vi "Ctrls state & value on Start-Stop.vi"(8 "error in (no error)":errorcluster, 11 "Queue data":T1) -> (0 "error out":errorcluster)   [LabVIEW 2020]
uses:
  Typedefs/Next state queue data.ctl
  Typedefs/Start-Stop Enum.ctl
  Typedefs/Top level VI states.ctl
  Typedefs/Read Write Enum.ctl
  Typedefs/Set Main VI cursor.ctl
  Global Variables/gl_UI Ctrl Refs.vi
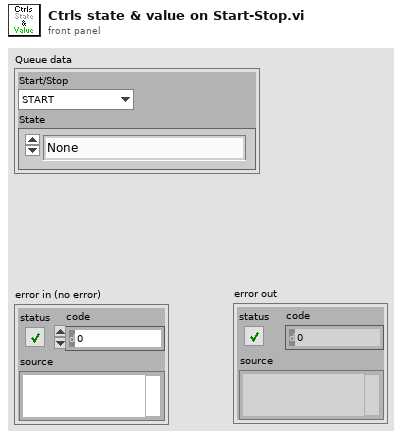
[diagram p1: front panel]
types:
  T1 = typedef "Next state queue data.ctl" = cluster{"Start/Stop":T2, "State":T3}
  T2 = typedef "Start-Stop Enum.ctl" = enum16{"START", "STOP"}
  T3 = typedef "Top level VI states.ctl" = enum16{"None", "Initialise UI", "<STACK PROTOCOL STATES>", "AOL Zstack-START", "AOL Zstack-STOP", "Motor Zstack-START", "Motor Zstack-STOP", "Parameter Sweep-START", "Parameter Sweep-STOP", "<ACQUISITION PROTOCOL STATES> ", "Functional Acquisition-START", "Functional Acquisition-STOP", "Single Plane Acquisition-START", "Single Plane Acquisition-STOP", "Volume Acquisition-START", "Volume Acquisition-STOP", "<LIVE IMAGING PROTOCOL STATES>", "Live Imaging-START", "Live Imaging-STOP", "Live Plane Imaging-START", "Live Plane Imaging-STOP", "Live Volume Imaging-START", "Live Volume Imaging-STOP", "<MOVEMENT CORRECTION PROTOCOL STATES>", "EXIT"}
  T4 = enum8{"Enabled", "Disabled", "Disabled and Grayed Out"}
  T5 = typedef "Read Write Enum.ctl" = enum16{"Read", "Write"}
  T6 = typedef "UI ctrl refs cluster.ctl" = cluster{"Top level VI path":path, "Top level VI ref":refnum<vi>, "User menu ref":refnum<k9>, "Sub Panel control":refnum<vi>, "Imaging Param Tab":refnum<vi>, "Occurrence-Start drivers":refnum<k4>, "Occurrence-Speed logging initialised":refnum<k4>, "Occurrence-XYZ stage initialised":refnum<k4>, "Exit button":refnum<vi>, "Status ind":refnum<vi>, "Set as origin":refnum<vi>, "Speed Logging":refnum<vi>, "Time Lapse":refnum<vi>, "Live Imaging":refnum<vi>, "AOL Z Stack":refnum<vi>, "Motor Z Stack":refnum<vi>, "Funct Acq button":refnum<vi>, "Hard Shutter":refnum<vi>, "Virtual Shutter":refnum<vi>, "Laser Power":refnum<vi>, "AOL Mode":refnum<vi>, "Frame Size":refnum<vi>, "Field of View":refnum<vi>, "Dwell Time":refnum<vi>, "Zoom":refnum<vi>, "AOL Z":refnum<vi>, "Objective":refnum<vi>, "Axis":refnum<vi>, "Paths & Names":refnum<vi>, "Experiment folder path (ind.)":refnum<vi>, "Last State (Ind.)":refnum<vi>, "Averages":refnum<vi>, "Angle (degrees)":refnum<vi>, "X centre":refnum<vi>, "Y centre":refnum<vi>, "Plane Mode":refnum<vi>, "# Planes":refnum<vi>, "Z Start":refnum<vi>, "Z Stop":refnum<vi>, "Z Step":refnum<vi>, "PMT 1":refnum<vi>, "PMT 2":refnum<vi>, "Stage XYZ Position":refnum<vi>, "Pockels@Z Start":refnum<vi>, "Pockels@Z Stop":refnum<vi>, "Obtain Z Start":refnum<vi>, "Obtain Z Stop":refnum<vi>, "Live stim.trig.period":refnum<vi>, "Live stim.trig.enable":refnum<vi>, "Movement Correction":refnum<vi>, "Load Reference Image":refnum<vi>, "XY Stage Move":refnum<vi>, "MovCor Cluster":refnum<vi>, "RefDAQParam":refnum<vi>, "Funct. Acq. Pockels Modulation":refnum<vi>, "Ref Laser Power":refnum<vi>, "Enable Video Recording":refnum<vi>, "Video Record-Live Imaging":refnum<vi>, "Video Record-Funct acq":refnum<vi>, "Reference Source":refnum<vi>, "AOL Z-stack Chirps Ready (ind)":refnum<vi>, "Target time between mov.cor. ref triggers (ms)":refnum<vi>, "Funct. Acq. Ref frame save":refnum<vi>, "Tracking button":refnum<vi>, "Show ref plots window":refnum<vi>, "Center freq ind (nm)":refnum<vi>, "Pickup mode (ind)":refnum<vi>, "Logging queue (ind)":refnum<vi>, "Back aperture power (ind.)":refnum<vi>, "Power after objective (ind.)":refnum<vi>, "Switch user":refnum<vi>, "Ls1 Conn. Status":refnum<vi>, "Ls1Tuning Status":refnum<vi>, "Ls1 Faults":refnum<vi>, "Ls1 Connection":refnum<vi>, "Ls1 Mode":refnum<vi>, "Ls1 POWER [mW]":refnum<vi>, "Ls1Shutter":refnum<vi>, "Ls1 Wavelength":refnum<vi>, "Ls1 Note":refnum<vi>, "Ls1 Confirm Wav":refnum<vi>, "Ls1 PreChrp Prism1":refnum<vi>, "Ls1 PreChrp Prism2":refnum<vi>, "Ls1 wav top Ind":refnum<vi>, "Ls1 power top Ind":refnum<vi>, "Ls1 Pump peak Hold":refnum<vi>, "Ls1 Status Ind":refnum<vi>, "Ls1 wav cancel":refnum<vi>, "Experiment Type":refnum<vi>, "Biology Information":refnum<vi>, "Camera recording status":refnum<vi>, "Optimise Obj. Pos.":refnum<vi>}
  T7 = typedef "Set Main VI cursor.ctl" = enum16{"Release busy cursor", "Set busy cursor"}
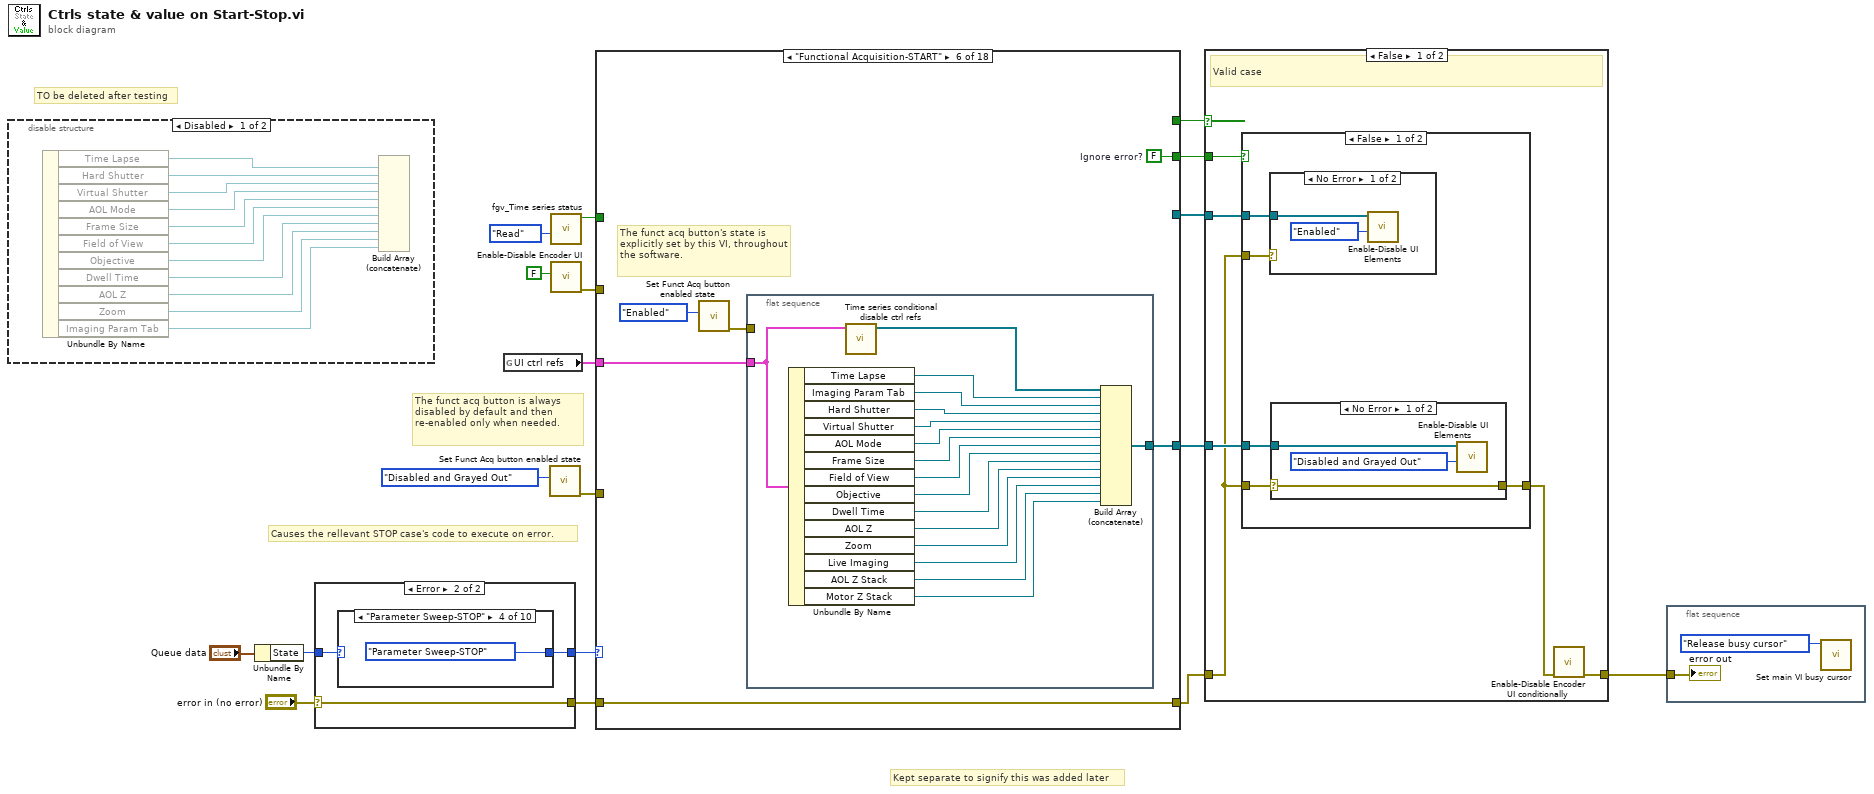
[diagram p0: block diagram]
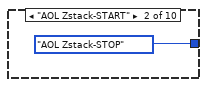
[diagram p5: hidden frame]
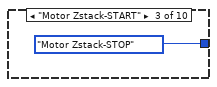
[diagram p6: hidden frame]
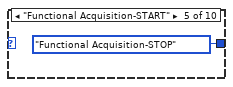
[diagram p7: hidden frame]
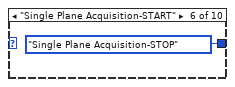
[diagram p8: hidden frame]
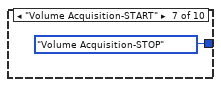
[diagram p9: hidden frame]
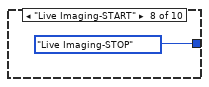
[diagram p10: hidden frame]
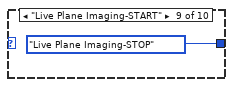
[diagram p11: hidden frame]
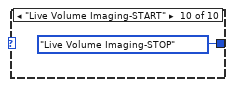
[diagram p12: hidden frame]
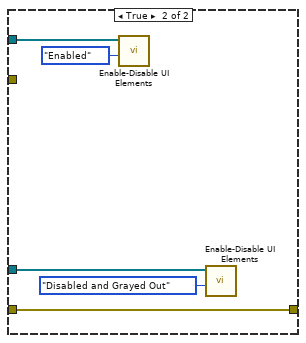
[diagram p15: hidden frame]
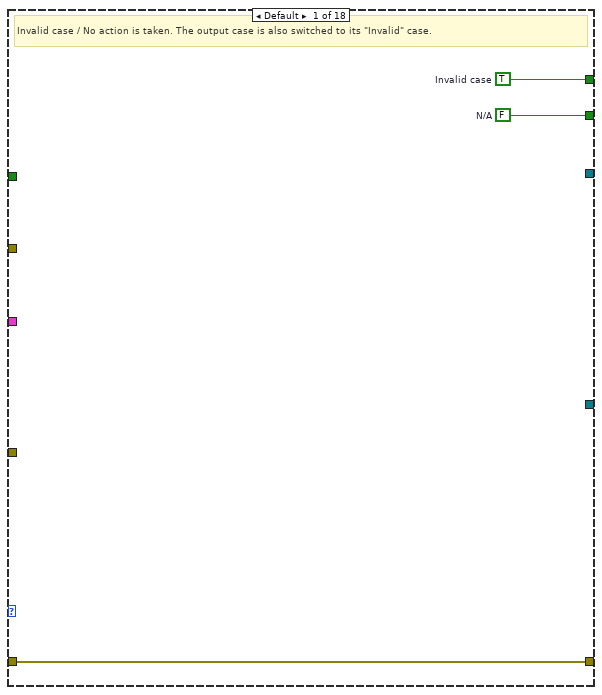
[diagram p17: hidden frame]
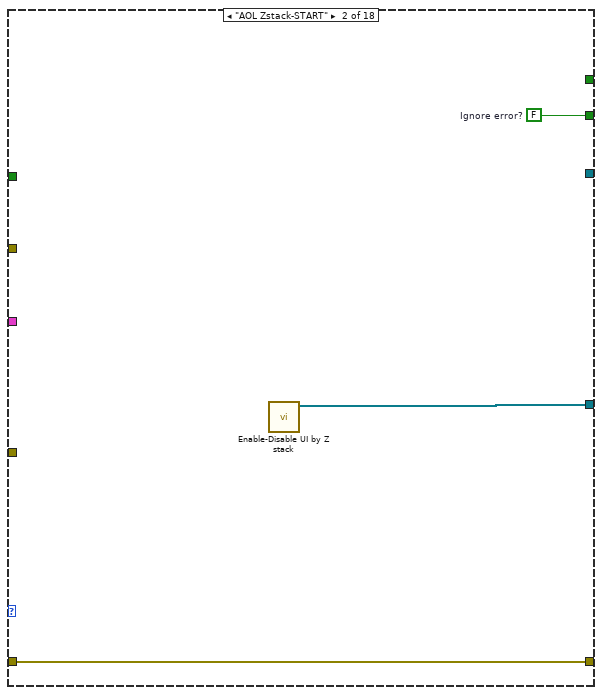
[diagram p18: hidden frame]
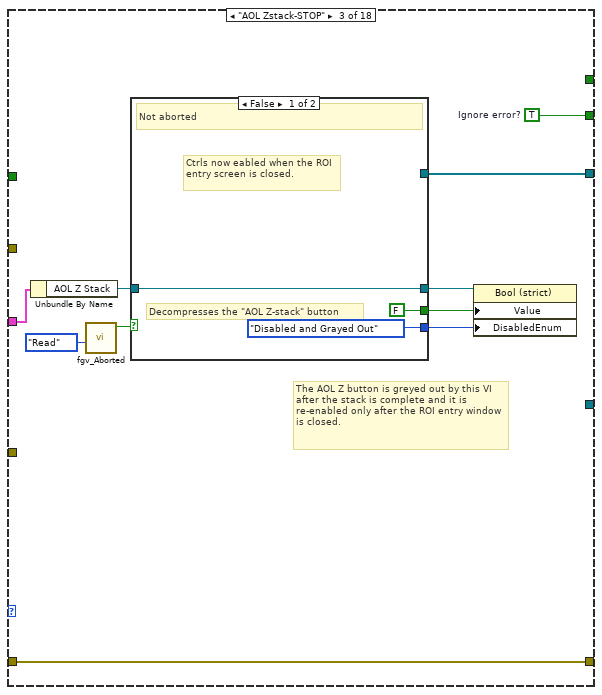
[diagram p19: hidden frame]
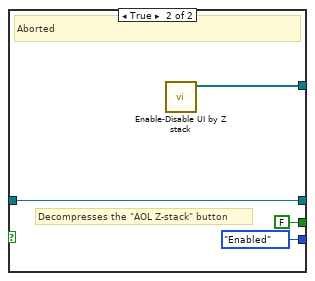
[diagram p20: hidden frame]
diagram:
  # "TO be deleted after testing"
  # "Kept separate to signify this was added later"
  # "The funct acq button is always disabled by default and then re-enabled only when needed."
  # "Causes the rellevant STOP case's code to execute on error."
  n1 = disable-structure shown="Disabled" {
    frame Disabled {
      n2 = Unbundle By Name() -> ("Time Lapse"=w20:refnum<vi>, "Hard Shutter"=w22:refnum<vi>, "Virtual Shutter"=w23:refnum<vi>, "AOL Mode"=w24:refnum<vi>, "Frame Size"=w25:refnum<vi>, "Field of View"=w26:refnum<vi>, "Objective"=w27:refnum<vi>, "Dwell Time"=w28:refnum<vi>, "AOL Z"=w29:refnum<vi>, "Zoom"=w30:refnum<vi>, "Imaging Param Tab"=w21:refnum<vi>)  [unwired: 1 in]
      n3 = Build Array (concatenate)(w20, w22, w23, w24, w25, w26, w27, w28, w29, w30, w21) -> (w19:refnum<vi>[])  [unwired: 1 out]
    }
    frame Enabled {
    }
  }
  n4 = Unbundle By Name("Queue data") -> ("State"=w10:T3)
  n5 = case shown="Error" "error in (no error)" {
    selector: "error in (no error)" -> [w31 w35]
    tunnel: w10 -> [w32 w34]
    tunnel: [w32 w33] -> w8
    tunnel: [w31 w35] -> w4
    frame No Error {
    }
    frame Error {
      n6 = case shown="\"Parameter Sweep-STOP\"" w34 {
        selector: w34 -> [w36 _ _ _ _ _ _ _ _ _]
        tunnel: [w36 Top_level_VI_states."AOL Zstack-STOP" ("State") Top_level_VI_states."Motor Zstack-STOP" ("State") Top_level_VI_states."Parameter Sweep-STOP" ("State") Top_level_VI_states."Functional Acquisition-STOP" ("State") Top_level_VI_states."Single Plane Acquisition-STOP" ("State") Top_level_VI_states."Volume Acquisition-STOP" ("State") Top_level_VI_states."Live Imaging-STOP" ("State") Top_level_VI_states."Live Plane Imaging-STOP" ("State") Top_level_VI_states."Live Volume Imaging-STOP" ("State")] -> w33
        frame Default {
        }
        frame "AOL Zstack-START" {
        }
        frame "Motor Zstack-START" {
        }
        frame "Parameter Sweep-STOP" {
        }
        frame "Functional Acquisition-START" {
        }
        frame "Single Plane Acquisition-START" {
        }
        frame "Volume Acquisition-START" {
        }
        frame "Live Imaging-START" {
        }
        frame "Live Plane Imaging-START" {
        }
        frame "Live Volume Imaging-START" {
        }
      }
    }
  }
  n7 = global read "gl_UI Ctrl Refs.vi" "UI ctrl refs"() -> (w18:T6)
  n8 = call "Set Funct Acq button enabled state.vi"("Disabled"=T4."Disabled and Grayed Out") -> ("error out"=w6:errorcluster)  [unwired: 10 in]
  n9 = call "fgv_Time series status.vi"("Function"=Read_Write_Enum."Read") -> ("Timelapse?"=w11:bool)  [unwired: 10 in]
  n10 = call "Enable-Disable Encoder UI.vi"("Cam VidRec.VidRec available"=FALSE) -> ("error out"=w1:errorcluster)  [unwired: 10 in]
  n11 = case "Message Cases" shown="\"Functional Acquisition-START\"" w8 {
    tunnel: w18 -> [_ _ w54 _ w73 w92 w113 w133 w152 w171 w189 w206 w227 w247 w264 w278 w296 w311]
    tunnel: [_ _ w57 _ w72 _ w123 _ w161 _ w187 _ w237 _ w268 _ w299 _] -> w17
    tunnel: [w48 _ _ _ _ _ _ _ _ _ _ _ _ _ _ _ _ _] -> w15
    tunnel: [_ w50 _ w71 _ w94 _ w142 _ w177 _ w216 _ w252 _ w283 _ w313] -> w14
    tunnel: [w47 w51 w61 w70 w81 w93 w122 w141 w160 w176 w205 w215 w236 w251 w267 w282 w298 w312] -> w13
    tunnel: w11 -> [_ _ _ _ _ _ _ _ _ _ _ w211 _ w250 _ w281 _ w310]
    tunnel: w6 -> [_ _ _ _ _ _ _ _ _ _ _ _ _ _ _ _ _ _]
    tunnel: w4 -> [w46 w49 w60 w69 w80 w89 w114 w134 w153 w172 w204 w207 w228 w248 w265 w279 w297 w309]
    tunnel: [w46 w49 w60 w69 w80 w89 w114 w134 w153 w172 w204 w207 w228 w248 w265 w279 w297 w309] -> w3
    tunnel: w1 -> [_ _ _ _ _ _ _ _ _ _ _ _ _ _ _ _ _ _]
    frame Default {
      w47 = FALSE  # N/A
      w48 = TRUE  # Invalid case
      # "Invalid case / No action is taken. The output case is also switched to its \"Invalid\" case."
    }
    frame "AOL Zstack-START" {
      w51 = FALSE  # Ignore error?
      n12 = call "Enable-Disable UI by Z stack.vi"() -> ("Controls refs to enable/disable"=w50:refnum<vi>[])  [unwired: 11 in]
    }
    frame "AOL Zstack-STOP" {
      w61 = TRUE  # Ignore error?
      # "The AOL Z button is greyed out by this VI after the stack is complete and it is re-enabled only after the ROI entry window is closed."
      n13 = Unbundle By Name(w54) -> ("AOL Z Stack"=w53:refnum<vi>)
      n14 = call "fgv_Aborted.vi"("Function"=Read_Write_Enum."Read") -> ("Funct Acq Aborted?"=w58:bool)  [unwired: 9 in, 1 out]
      n15 = case shown="False" w58 {
        tunnel: [_ w68] -> w57
        tunnel: [FALSE ("Value") FALSE ("Value")] -> w56
        tunnel: [T4."Disabled and Grayed Out" ("Disabled") T4."Enabled" ("Disabled")] -> w55
        tunnel: w53 -> [w63 w67]
        tunnel: [w63 w67] -> w52
        frame False {
          # "Ctrls now eabled when the ROI entry screen is closed."
          # "Decompresses the \"AOL Z-stack\" button"
          # "Not aborted"
        }
        frame True {
          # "Decompresses the \"AOL Z-stack\" button"
          # "Aborted"
          n16 = call "Enable-Disable UI by Z stack.vi"() -> ("Controls refs to enable/disable"=w68:refnum<vi>[])  [unwired: 11 in]
        }
      }
      n17 = property class="Bool (strict)"(reference=w52, "Value"=w56, "DisabledEnum"=w55) -> ()  [unwired: 1 in, 2 out]
    }
    frame "Motor Zstack-START" {
      w70 = FALSE  # Ignore error?
      n18 = call "Enable-Disable UI by Motor Z stack.vi"() -> ("Controls to disable"=w71:refnum<vi>[])  [unwired: 11 in]
    }
    frame "Motor Zstack-STOP" {
      w81 = TRUE  # Ignore error?
      # "The Motor Z button is greyed out by this VI after the stack is complete and it is re-enabled only after the ROI entry window is closed."
      n19 = Unbundle By Name(w73) -> ("Motor Z Stack"=w78:refnum<vi>)
      n20 = call "fgv_Aborted.vi"("Function"=Read_Write_Enum."Read") -> ("Funct Acq Aborted?"=w75:bool)  [unwired: 9 in, 1 out]
      n21 = case shown="True" w75 {
        tunnel: [_ w85] -> w72
        tunnel: [FALSE ("Value") FALSE ("Value")] -> w76
        tunnel: [T4."Disabled and Grayed Out" ("Disabled") T4."Enabled" ("Disabled")] -> w77
        tunnel: w78 -> [w83 w88]
        tunnel: [w83 w88] -> w79
        frame False {
          # "Ctrls now eabled when the ROI entry screen is closed."
          # "Decompresses the \"AOL Z-stack\" button"
          # "Not aborted"
        }
        frame True {
          # "Decompresses the \"Motor Z-stack\" button"
          # "Aborted"
          n22 = call "Enable-Disable UI by Motor Z stack.vi"() -> ("Controls to disable"=w85:refnum<vi>[])  [unwired: 11 in]
        }
      }
      n23 = property class="Bool (strict)"(reference=w79, "Value"=w76, "DisabledEnum"=w77) -> ()  [unwired: 1 in, 2 out]
    }
    frame "Functional Acquisition-START" {
      w93 = FALSE  # Ignore error?
      # "The funct acq button's state is explicitly set by this VI, throughout the software."
      n24 = call "Set Funct Acq button enabled state.vi"("Disabled"=T4."Enabled") -> ("error out"=w90:errorcluster)  [unwired: 10 in]
      n25 = flat-sequence {
        tunnel: [w111] -> w94
        tunnel: w92 -> [w95]
        tunnel: w90 -> [_]
        frame #0 {
          n26 = Unbundle By Name(w95) -> ("Time Lapse"=w100:refnum<vi>, "Imaging Param Tab"=w101:refnum<vi>, "Hard Shutter"=w102:refnum<vi>, "Virtual Shutter"=w103:refnum<vi>, "AOL Mode"=w104:refnum<vi>, "Frame Size"=w105:refnum<vi>, "Field of View"=w106:refnum<vi>, "Objective"=w107:refnum<vi>, "Dwell Time"=w108:refnum<vi>, "AOL Z"=w109:refnum<vi>, "Zoom"=w110:refnum<vi>, "Live Imaging"=w98:refnum<vi>, "AOL Z Stack"=w97:refnum<vi>, "Motor Z Stack"=w96:refnum<vi>)
          n27 = call "Time series conditional disable ctrl refs.vi"("UI ctrl refs"=w95) -> ("Ctrl refs"=w99:refnum<vi>[])  [unwired: 10 in]
          n28 = Build Array (concatenate)(w99, w100, w101, w102, w103, w104, w105, w106, w107, w108, w109, w110, w98, w97, w96) -> (w111:refnum<vi>[])
        }
      }
    }
    frame "Functional Acquisition-STOP" {
      w122 = TRUE  # Ignore error?
      # "Decompresses the \"funct. acq.\" button"
      # "Controls enabled when Live Imaging is stopped"
      n29 = Unbundle By Name(w113) -> ("Time Lapse"=w120:refnum<vi>, "Hard Shutter"=w124:refnum<vi>, "Virtual Shutter"=w125:refnum<vi>, "AOL Mode"=w126:refnum<vi>, "Frame Size"=w127:refnum<vi>, "Field of View"=w128:refnum<vi>, "Objective"=w129:refnum<vi>, "Dwell Time"=w130:refnum<vi>, "AOL Z"=w131:refnum<vi>, "Zoom"=w132:refnum<vi>, "Imaging Param Tab"=w121:refnum<vi>, "Live Imaging"=w119:refnum<vi>, "AOL Z Stack"=w118:refnum<vi>, "Motor Z Stack"=w117:refnum<vi>)
      n30 = call "Time series conditional disable ctrl refs.vi"("UI ctrl refs"=w113) -> ("Ctrl refs"=w112:refnum<vi>[])  [unwired: 10 in]
      n31 = call "Set Funct Acq button value.vi"("Functional Acquisition button's new value"=FALSE ("Value")) -> ()  [unwired: 10 in, 1 out]
      n32 = call "Set Funct Acq button enabled state.vi"("Disabled"=T4."Enabled") -> ()  [unwired: 10 in, 1 out]
      n33 = Build Array (concatenate)(w120, w124, w125, w126, w127, w128, w129, w130, w131, w132, w121, w119, w118, w117, w112) -> (w123:refnum<vi>[])
    }
    frame "Single Plane Acquisition-START" {
      w141 = FALSE  # Ignore error?
      # "Not in use - placeholder only"
      n34 = Unbundle By Name(w133) -> ("Time Lapse"=w139:refnum<vi>, "Imaging Param Tab"=w140:refnum<vi>, "Hard Shutter"=w143:refnum<vi>, "Virtual Shutter"=w144:refnum<vi>, "AOL Mode"=w145:refnum<vi>, "Frame Size"=w146:refnum<vi>, "Field of View"=w147:refnum<vi>, "Objective"=w148:refnum<vi>, "Dwell Time"=w149:refnum<vi>, "AOL Z"=w150:refnum<vi>, "Zoom"=w151:refnum<vi>, "AOL Z Stack"=w137:refnum<vi>, "Motor Z Stack"=w136:refnum<vi>, "Live Imaging"=w135:refnum<vi>)
      n35 = call "Time series conditional disable ctrl refs.vi"("UI ctrl refs"=w133) -> ("Ctrl refs"=w138:refnum<vi>[])  [unwired: 10 in]
      n36 = Build Array (concatenate)(w138, w139, w140, w143, w144, w145, w146, w147, w148, w149, w150, w151, w137, w136, w135) -> (w142:refnum<vi>[])
    }
    frame "Single Plane Acquisition-STOP" {
      w160 = TRUE  # Ignore error?
      # "Not in use place holder only"
      n37 = Unbundle By Name(w152) -> ("Time Lapse"=w158:refnum<vi>, "Hard Shutter"=w162:refnum<vi>, "Virtual Shutter"=w163:refnum<vi>, "AOL Mode"=w164:refnum<vi>, "Frame Size"=w165:refnum<vi>, "Field of View"=w166:refnum<vi>, "Objective"=w167:refnum<vi>, "Dwell Time"=w168:refnum<vi>, "AOL Z"=w169:refnum<vi>, "Zoom"=w170:refnum<vi>, "Imaging Param Tab"=w159:refnum<vi>, "AOL Z Stack"=w157:refnum<vi>, "Motor Z Stack"=w156:refnum<vi>, "Live Imaging"=w155:refnum<vi>)
      n38 = call "Time series conditional disable ctrl refs.vi"("UI ctrl refs"=w152) -> ("Ctrl refs"=w154:refnum<vi>[])  [unwired: 10 in]
      n39 = Build Array (concatenate)(w154, w158, w162, w163, w164, w165, w166, w167, w168, w169, w170, w159, w157, w156, w155) -> (w161:refnum<vi>[])
    }
    frame "Volume Acquisition-START" {
      w176 = FALSE  # Ignore error?
      # "Not in use place holder only"
      n40 = Unbundle By Name(w171) -> ("Time Lapse"=w174:refnum<vi>, "Imaging Param Tab"=w175:refnum<vi>, "Hard Shutter"=w178:refnum<vi>, "Virtual Shutter"=w179:refnum<vi>, "AOL Mode"=w180:refnum<vi>, "Frame Size"=w181:refnum<vi>, "Field of View"=w182:refnum<vi>, "Objective"=w183:refnum<vi>, "Dwell Time"=w184:refnum<vi>, "AOL Z"=w185:refnum<vi>, "Zoom"=w186:refnum<vi>)
      n41 = call "Time series conditional disable ctrl refs.vi"("UI ctrl refs"=w171) -> ("Ctrl refs"=w173:refnum<vi>[])  [unwired: 10 in]
      n42 = Build Array (concatenate)(w173, w174, w175, w178, w179, w180, w181, w182, w183, w184, w185, w186) -> (w177:refnum<vi>[])
    }
    frame "Volume Acquisition-STOP" {
      w205 = TRUE  # Ignore error?
      # "Not in use place holder only"
      n43 = call "Time series conditional disable ctrl refs.vi"("UI ctrl refs"=w189) -> ("Ctrl refs"=w188:refnum<vi>[])  [unwired: 10 in]
      n44 = Unbundle By Name(w189) -> ("Time Lapse"=w193:refnum<vi>, "Hard Shutter"=w195:refnum<vi>, "Virtual Shutter"=w196:refnum<vi>, "AOL Mode"=w197:refnum<vi>, "Frame Size"=w198:refnum<vi>, "Field of View"=w199:refnum<vi>, "Objective"=w200:refnum<vi>, "Dwell Time"=w201:refnum<vi>, "AOL Z"=w202:refnum<vi>, "Zoom"=w203:refnum<vi>, "Imaging Param Tab"=w194:refnum<vi>, "Live Imaging"=w192:refnum<vi>, "AOL Z Stack"=w191:refnum<vi>, "Motor Z Stack"=w190:refnum<vi>)
      n45 = Build Array (concatenate)(w188, w193, w195, w196, w197, w198, w199, w200, w201, w202, w203, w194, w192, w191, w190) -> (w187:refnum<vi>[])
    }
    frame "Live Imaging-START" {
      w215 = FALSE  # Ignore error?
      # "<-- Allowed"
      # "<-- Allowed"
      n46 = case shown="False" w211 {
        tunnel: w206 -> [_ w226]
        tunnel: [_ w225] -> w212
        frame False {
          # "Re-enable the Speed logging tick box"
          # "Timelapse is not ON"
          n47 = call "Enable-Disable Encoder UI conditionally.vi"() -> ()  [unwired: 11 in, 1 out]
        }
        frame True {
          # "Time-lapse is ON"
          n48 = call "Time series conditional disable ctrl refs.vi"("UI ctrl refs"=w226) -> ("Ctrl refs"=w225:refnum<vi>[])  [unwired: 10 in]
        }
      }
      n49 = Unbundle By Name(w206) -> ("Hard Shutter"=w210:refnum<vi>, "Virtual Shutter"=w217:refnum<vi>, "AOL Mode"=w218:refnum<vi>, "Frame Size"=w219:refnum<vi>, "Field of View"=w220:refnum<vi>, "Objective"=w221:refnum<vi>, "Dwell Time"=w222:refnum<vi>, "AOL Z"=w223:refnum<vi>, "Zoom"=w224:refnum<vi>, "AOL Z Stack"=w214:refnum<vi>, "Motor Z Stack"=w213:refnum<vi>, "Movement Correction"=w209:refnum<vi>, "Load Reference Image"=w208:refnum<vi>)  [unwired: 2 out]
      n50 = Build Array (concatenate)(w212, w210, w217, w218, w219, w220, w221, w222, w223, w224, w214, w213, w209, w208) -> (w216:refnum<vi>[])
    }
    frame "Live Imaging-STOP" {
      w236 = TRUE  # Ignore error?
      # "<-- Allowed"
      # "Decompresses the \"Live Imaging.\" button"
      # "<-- Allowed"
      n51 = Unbundle By Name(w227) -> ("Hard Shutter"=w238:refnum<vi>, "Virtual Shutter"=w239:refnum<vi>, "AOL Mode"=w240:refnum<vi>, "Frame Size"=w241:refnum<vi>, "Field of View"=w242:refnum<vi>, "Objective"=w243:refnum<vi>, "Dwell Time"=w244:refnum<vi>, "AOL Z"=w245:refnum<vi>, "Zoom"=w246:refnum<vi>, "AOL Z Stack"=w235:refnum<vi>, "Motor Z Stack"=w234:refnum<vi>, "Movement Correction"=w231:refnum<vi>, "Load Reference Image"=w230:refnum<vi>)  [unwired: 2 out]
      n52 = Unbundle By Name(w227) -> ("Live Imaging"=w233:refnum<vi>)
      n53 = call "Time series conditional disable ctrl refs.vi"("UI ctrl refs"=w227) -> ("Ctrl refs"=w229:refnum<vi>[])  [unwired: 10 in]
      n54 = property class="Bool (strict)"(reference=w233, "Value"=FALSE) -> ()  [unwired: 1 in, 2 out]
      n55 = Build Array (concatenate)(w229, w238, w239, w240, w241, w242, w243, w244, w245, w246, w235, w234, w231, w230) -> (w237:refnum<vi>[])
    }
    frame "Live Plane Imaging-START" {
      w251 = FALSE  # Ignore error?
      # "Not in use place holder only"
      n56 = case shown="True" w250 {
        tunnel: w247 -> [_ w263]
        tunnel: [_ w262] -> w249
        frame False {
          # "Re-enable the Speed logging tick box"
          # "Timelapse is not ON"
          n57 = call "Enable-Disable Encoder UI conditionally.vi"() -> ()  [unwired: 11 in, 1 out]
        }
        frame True {
          # "Time-lapse is ON"
          n58 = call "Time series conditional disable ctrl refs.vi"("UI ctrl refs"=w263) -> ("Ctrl refs"=w262:refnum<vi>[])  [unwired: 10 in]
        }
      }
      n59 = Unbundle By Name(w247) -> ("Hard Shutter"=w253:refnum<vi>, "Virtual Shutter"=w254:refnum<vi>, "AOL Mode"=w255:refnum<vi>, "Frame Size"=w256:refnum<vi>, "Field of View"=w257:refnum<vi>, "Objective"=w258:refnum<vi>, "Dwell Time"=w259:refnum<vi>, "AOL Z"=w260:refnum<vi>, "Zoom"=w261:refnum<vi>)
      n60 = Build Array (concatenate)(w249, w253, w254, w255, w256, w257, w258, w259, w260, w261) -> (w252:refnum<vi>[])
    }
    frame "Live Plane Imaging-STOP" {
      w267 = TRUE  # Ignore error?
      # "Not in use place holder only"
      n61 = Unbundle By Name(w264) -> ("Hard Shutter"=w269:refnum<vi>, "Virtual Shutter"=w270:refnum<vi>, "AOL Mode"=w271:refnum<vi>, "Frame Size"=w272:refnum<vi>, "Field of View"=w273:refnum<vi>, "Objective"=w274:refnum<vi>, "Dwell Time"=w275:refnum<vi>, "AOL Z"=w276:refnum<vi>, "Zoom"=w277:refnum<vi>)
      n62 = call "Time series conditional disable ctrl refs.vi"("UI ctrl refs"=w264) -> ("Ctrl refs"=w266:refnum<vi>[])  [unwired: 10 in]
      n63 = Build Array (concatenate)(w266, w269, w270, w271, w272, w273, w274, w275, w276, w277) -> (w268:refnum<vi>[])
    }
    frame "Live Volume Imaging-START" {
      w282 = FALSE  # Ignore error?
      # "Not in use place holder only"
      n64 = Unbundle By Name(w278) -> ("Hard Shutter"=w284:refnum<vi>, "Virtual Shutter"=w285:refnum<vi>, "AOL Mode"=w286:refnum<vi>, "Frame Size"=w287:refnum<vi>, "Field of View"=w288:refnum<vi>, "Objective"=w289:refnum<vi>, "Dwell Time"=w290:refnum<vi>, "AOL Z"=w291:refnum<vi>, "Zoom"=w292:refnum<vi>)
      n65 = case shown="False" w281 {
        tunnel: w278 -> [_ w294]
        tunnel: [_ w293] -> w280
        frame False {
          # "Re-enable the Speed logging tick box"
          # "Time-lapse is not ON"
          n66 = call "Enable-Disable Encoder UI conditionally.vi"() -> ()  [unwired: 11 in, 1 out]
        }
        frame True {
          # "Time-lapse is ON"
          n67 = call "Time series conditional disable ctrl refs.vi"("UI ctrl refs"=w294) -> ("Ctrl refs"=w293:refnum<vi>[])  [unwired: 10 in]
        }
      }
      n68 = Build Array (concatenate)(w280, w284, w285, w286, w287, w288, w289, w290, w291, w292) -> (w283:refnum<vi>[])
    }
    frame "Live Volume Imaging-STOP" {
      w298 = TRUE  # Ignore error?
      # "Not in use place holder only"
      n69 = Unbundle By Name(w296) -> ("Hard Shutter"=w300:refnum<vi>, "Virtual Shutter"=w301:refnum<vi>, "AOL Mode"=w302:refnum<vi>, "Frame Size"=w303:refnum<vi>, "Field of View"=w304:refnum<vi>, "Objective"=w305:refnum<vi>, "Dwell Time"=w306:refnum<vi>, "AOL Z"=w307:refnum<vi>, "Zoom"=w308:refnum<vi>)
      n70 = call "Time series conditional disable ctrl refs.vi"("UI ctrl refs"=w296) -> ("Ctrl refs"=w295:refnum<vi>[])  [unwired: 10 in]
      n71 = Build Array (concatenate)(w300, w301, w302, w303, w304, w305, w306, w307, w308, w295) -> (w299:refnum<vi>[])
    }
    frame "EXIT" {
      w312 = FALSE  # Ignore error?
      n72 = disable-structure shown="Disabled" {
        disable-tunnel: [w322 _] -> w313
        disable-tunnel: w311 -> [w319 _]
        disable-tunnel: w310 -> [w317 _]
        frame Disabled {
          # "<-- Allowed"
          # "<-- Allowed"
          # "Controls disabled during Live Imaging"
          n73 = case shown="False" w317 {
            tunnel: w319 -> [_ w332]
            tunnel: [_ w331] -> w318
            frame False {
              # "Re-enable the Speed logging tick box"
              # "Time-lapse is not ON"
              n74 = call "Enable-Disable Encoder UI conditionally.vi"() -> ()  [unwired: 11 in, 1 out]
            }
            frame True {
              # "Time-lapse is ON"
              n75 = call "Time series conditional disable ctrl refs.vi"("UI ctrl refs"=w332) -> ("Ctrl refs"=w331:refnum<vi>[])  [unwired: 10 in]
            }
          }
          n76 = Unbundle By Name(w319) -> ("Hard Shutter"=w316:refnum<vi>, "Virtual Shutter"=w323:refnum<vi>, "AOL Mode"=w324:refnum<vi>, "Frame Size"=w325:refnum<vi>, "Field of View"=w326:refnum<vi>, "Objective"=w327:refnum<vi>, "Dwell Time"=w328:refnum<vi>, "AOL Z"=w329:refnum<vi>, "Zoom"=w330:refnum<vi>, "AOL Z Stack"=w321:refnum<vi>, "Motor Z Stack"=w320:refnum<vi>, "Movement Correction"=w315:refnum<vi>, "Load Reference Image"=w314:refnum<vi>)  [unwired: 2 out]
          n77 = Build Array (concatenate)(w318, w316, w323, w324, w325, w326, w327, w328, w329, w330, w321, w320, w315, w314) -> (w322:refnum<vi>[])
        }
        frame Enabled {
        }
      }
    }
  }
  n78 = case shown="False" w15 {
    tunnel: w17 -> [w338 _]
    tunnel: w14 -> [w337 _]
    tunnel: w13 -> [w336 _]
    tunnel: w3 -> [w334 w355]
    tunnel: [w335 w355] -> w5
    frame False {
      # "Valid case"
      n79 = case shown="False" w336 {
        tunnel: w334 -> [w343 _]
        tunnel: w338 -> [w342 w354]
        tunnel: w337 -> [w341 w353]
        tunnel: w334 -> [w340 w350]
        tunnel: [w339 w350] -> w333
        frame False {
          n80 = case shown="No Error" w343 {
            tunnel: w342 -> [w349 _]
            frame No Error {
              n81 = call "Enable-Disable UI Elements.vi"("Enable/Disable"=T4."Enabled", "Ctrl ref's"=w349) -> ()  [unwired: 9 in, 1 out]
            }
            frame Error {
            }
          }
          n82 = case shown="No Error" w340 {
            selector: w340 -> [w344 w347]
            tunnel: w341 -> [w346 _]
            tunnel: [w344 w347] -> w339
            frame No Error {
              n83 = call "Enable-Disable UI Elements.vi"("Enable/Disable"=T4."Disabled and Grayed Out", "Ctrl ref's"=w346) -> ()  [unwired: 9 in, 1 out]
            }
            frame Error {
            }
          }
        }
        frame True {
          n84 = call "Enable-Disable UI Elements.vi"("Enable/Disable"=T4."Enabled", "Ctrl ref's"=w354) -> ()  [unwired: 9 in, 1 out]
          n85 = call "Enable-Disable UI Elements.vi"("Enable/Disable"=T4."Disabled and Grayed Out", "Ctrl ref's"=w353) -> ()  [unwired: 9 in, 1 out]
        }
      }
      n86 = call "Enable-Disable Encoder UI conditionally.vi"("error in"=w333) -> ("error out"=w335:errorcluster)  [unwired: 10 in]
    }
    frame True {
      # "Invalid case"
    }
  }
  n87 = flat-sequence {
    tunnel: w5 -> [w356]
    frame #0 {
      n88 = call "Set main VI busy cursor.vi"("Main VI's cursor"=Set_Main_VI_cursor."Release busy cursor") -> ()  [unwired: 10 in, 1 out]
      "error out" <- w356
    }
  }
